vi "PH_Switch.read DB.vi"(1 "DB Entry to read":string, 5 "error in (no error)":errorcluster) -> (15 "Tagnames":T1={"Switch"="N/A", "True"="N/A", "False"="N/A"}, 16 "Beckhoff Instance":string, 17 "Captions":cluster{"True":string, "False":string}, 18 "Default Value":string, 19 "error out":errorcluster)   [LabVIEW 2014, in "PH_Switch.lvlib"]
doc: "This VI reads the database and stores the inform,ation to own attributes."
uses:
  PH_Switch.lvlib
  PH_Basics/PH_Common/PH_Common.lvlib
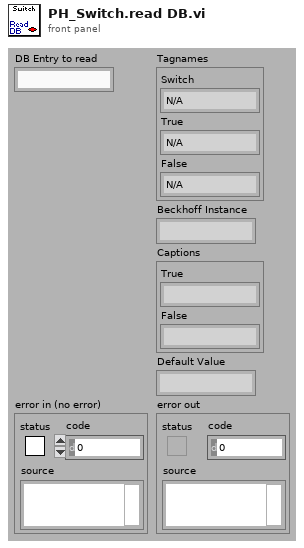
[diagram p1: front panel]
types:
  T1 = cluster{"Switch":string, "True":string, "False":string}
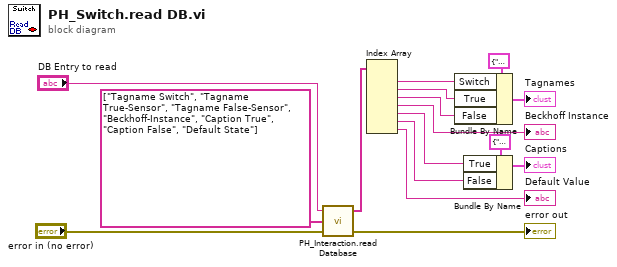
[diagram p0: block diagram]
diagram:
  n1 = call "PH_Interaction.read Database.vi"("error in (no error)"="error in (no error)", "Strings to search for"=string[] ["Tagname Switch", "Tagname True-Sensor", "Tagname False-Sensor", "Beckhoff-Instance", "Caption True", "Caption False", "Default State"], "DB Entry to read"="DB Entry to read") -> ("error out"=→"error out":errorcluster, "Values"=w12:string[])  [unwired: 1 in]
  n2 = Index Array(array=w12) -> (element #1=w6:string, element #2=w5:string, element #3=w4:string, element #4=→"Beckhoff Instance":string, element #5=w2:string, element #6=w1:string, element #7=→"Default Value":string)  [unwired: 7 in]
  n3 = Bundle By Name(cluster=T1 {"Switch"="N/A", "True"="N/A", "False"="N/A"} ("Tagnames"), "Switch"=w6, "True"=w5, "False"=w4) -> (→"Tagnames":T1)
  n4 = Bundle By Name(cluster=cluster{"True":string, "False":string} {"True"="", "False"=""} ("Captions"), "True"=w2, "False"=w1) -> (→"Captions":cluster{"True":string, "False":string})
